vi "Top Level Module.vi"() -> ()   [LabVIEW 2020]
uses:
  Classes/Sine/Sine.lvclass/Sine.ctl
  Classes/Sine/Sine.lvclass
  C:/Users/venug/Desktop/LV Test/LV-SOLID-base/LV-SOLID/SOLID Principles Demo/Interfaces/Sinusoid/Sinusoid.lvclass
panel:
  in  "Use Interface Caller?":bool
  in  "A":dbl
  in  "T":dbl
  in  "Phi":dbl
  out "y":dbl
  in  "t":dbl
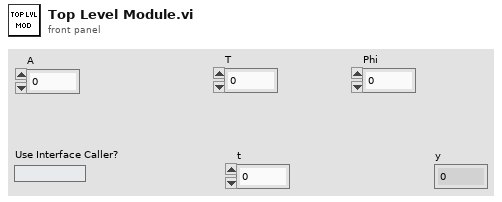
[diagram p1: front panel]
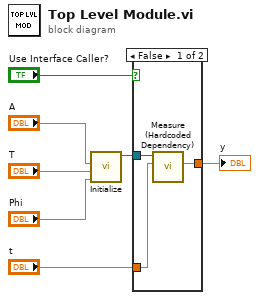
[diagram p0: block diagram]
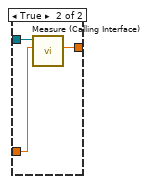
[diagram p2: hidden frame]
diagram:
  n1 = call "Initialize.vi"("Phi"="Phi", "T"="T", "A"="A") -> ("Sine out"=w7:refnum<class "Sine.lvclass">)  [unwired: 8 in]
  n2 = case shown="False" "Use Interface Caller?" {
    tunnel: w7 -> [w10 w13]
    tunnel: "t" -> [w9 w12]
    tunnel: [w8 w11] -> w5
    frame False {
      n3 = call "Measure (Hardcoded Dependency).vi"("t"=w9, "Sine in"=w10) -> ("y"=w8:dbl)  [unwired: 9 in]
    }
    frame True {
      n4 = call "Measure (Calling Interface).vi"("t"=w12, "Sinusoid in"=w13) -> ("y"=w11:dbl)  [unwired: 9 in]
    }
  }
  "y" <- w5
